vi "Move Cursor into ROI.vi"(8 "error in (no error)":errorcluster, 11 "Base Graph in":refnum<class "Base Graph.lvclass">) -> (0 "error out":errorcluster, 3 "Base Graph out":refnum<class "Base Graph.lvclass">)   [LabVIEW 2023, in "Base Graph.lvclass"]
uses:
  Base Graph.lvclass
  Base Graph.lvclass/Base Graph.ctl
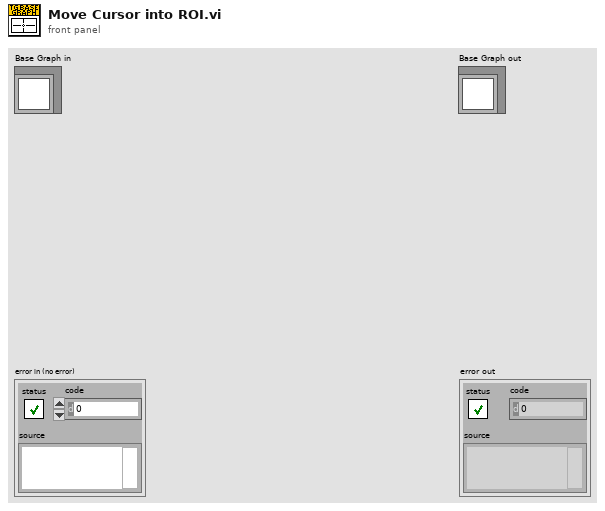
[diagram p1: front panel]
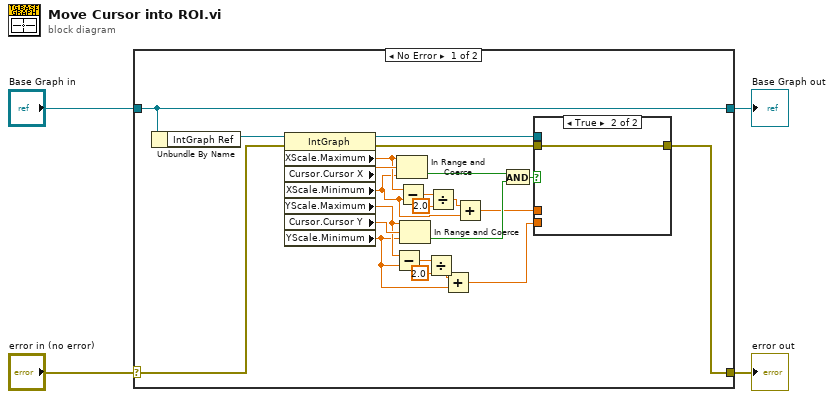
[diagram p0: block diagram]
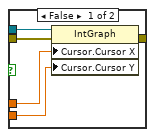
[diagram p2: hidden frame]
diagram:
  n1 = case shown="No Error" "error in (no error)" {
    selector: "error in (no error)" -> [w25 w35]
    tunnel: [w14 w35] -> w3
    tunnel: [w27 w34] -> w1
    tunnel: "Base Graph in" -> [w27 w34]
    frame No Error {
      n2 = Unbundle By Name(w27) -> ("IntGraph Ref"=w26:refnum<vi>)
      n3 = property class="IntGraph"(reference=w26, error in=w25) -> (reference out=w21:refnum<vi>, error out=w20:errorcluster, "XScale.Maximum"=w23:dbl, "Cursor.Cursor X"=w24:dbl, "XScale.Minimum"=w10:dbl, "YScale.Maximum"=w17:dbl, "Cursor.Cursor Y"=w18:dbl, "YScale.Minimum"=w13:dbl)
      n4 = Subtract(x=w17, y=w13) -> (x-y=w16:dbl)
      n5 = In Range and Coerce(upper limit=w23, x=w24, lower limit=w10) -> (In Range?=w7:bool)  [unwired: 1 out]
      n6 = Subtract(x=w23, y=w10) -> (x-y=w19:dbl)
      n7 = In Range and Coerce(upper limit=w17, x=w18, lower limit=w13) -> (In Range?=w8:bool)  [unwired: 1 out]
      n8 = Divide(x=w16, y=2.0) -> (x/y=w12:dbl)
      n9 = Divide(x=w19, y=2.0) -> (x/y=w11:dbl)
      n10 = Add(x=w12, y=w13) -> (x+y=w5:dbl)
      n11 = Add(x=w11, y=w10) -> (x+y=w6:dbl)
      n12 = And(x=w7, y=w8) -> (x .and. y?=w9:bool)
      n13 = case shown="True" w9 {
        tunnel: w21 -> [w32 _]
        tunnel: w20 -> [w31 w33]
        tunnel: [w30 w33] -> w14
        tunnel: w6 -> [w29 _]
        tunnel: w5 -> [w28 _]
        frame False {
          n14 = property class="IntGraph"(reference=w32, error in=w31, "Cursor.Cursor X"=w29, "Cursor.Cursor Y"=w28) -> (error out=w30:errorcluster)  [unwired: 1 out]
        }
        frame True {
        }
      }
    }
    frame Error {
    }
  }
  "error out" <- w3
  "Base Graph out" <- w1
